vi "Process.vi"(8 "error in":errorcluster, 11 "Lockin.UI":refnum<class "Instrument.Lockin.UI.lvclass">) -> (0 "error out":errorcluster, 3 "Lockin.UI out":refnum<class "Instrument.Lockin.UI.lvclass">)   [LabVIEW 2016, in "Instrument.Lockin.UI.lvclass"]
doc: "---------------------------------------------------------------\nJKI State Machine Objects™\nhttp://jki.net/state-machine-objects/\nCopyright (C) 2005-2015, JKI <info@jki.net>\nALL RIGHTS RESERVEDJKI State Machine Objects (SMO) 1.0.0.5\nJKI - JKI\nCopyright (c) 2016, JKI"
uses:
  Instrument.Lockin.UI.lvclass
  <vilib>/JKI/JKI SMO/SMO/SMO.lvclass
  <vilib>/JKI/JKI SMO/SMO/Typedefs/Parent Call--Enum.ctl
  <vilib>/JKI/JKI SMO/SMO.UI/SMO.UI.lvclass
  <userlib>/LevyLab/Levylab Instruments/SMOs/Instrument/Instrument.lvclass
  Instrument.Lockin/Typedefs/Lockin.getAll--Cluster.ctl
  Instrument.Lockin/Instrument.Lockin.lvclass
  <userlib>/LevyLab/Levylab Instruments/SMOs/Instrument UI/Instrument UI.lvclass
  C:/Program Files (x86)/National Instruments/LabVIEW 2016/user.lib/LevyLab/Levylab Instruments/SMOs/Instrument UI/Instrument UI.lvclass
  C:/Program Files (x86)/National Instruments/LabVIEW 2016/vi.lib/JKI/JKI SMO/SMO.UI/SMO.UI.lvclass
  C:/Program Files (x86)/National Instruments/LabVIEW 2016/vi.lib/JKI/JKI SMO/SMO/SMO.lvclass
  Typedefs/Y Axis Input-Enum.ctl
  Typedefs/X Axis-Enum.ctl
  Typedefs/Y Axis Output-Enum.ctl
  Typedefs/Display-Enum.ctl
  Lockin.DAQ/Typedefs/Function-enum.ctl
  Lockin.DAQ/Lockin.DAQ.lvclass
  Lockin.DAQ/Typedefs/REF-cluster.ctl
  Lockin.DAQ/Typedefs/AI Simulation-enum.ctl
  Lockin.DAQ/Typedefs/DAQType-enum.ctl
  Lockin.DAQ/Typedefs/Sampling.ctl
  Instrument.Lockin/Typedefs/Sample Mode--Enum.ctl
  Lockin.DAQ/Typedefs/446xAI-enum.ctl
  Lockin.DAQ/Typedefs/AI.coupling-enum.ctl
  Lockin.DAQ/Typedefs/446xAO-enum.ctl
  Typedefs/Device Configuration--Cluster.ctl
  Lockin.DAQ/Typedefs/Sweep Pattern--Enum.ctl
  <vilib>/JKI/JKI SMO/SMO/Typedefs/SMOState --Enum.ctl
  Lockin.DAQ/Typedefs/Cal Info - Cluster.ctl
  Typedefs/AO Channel--Cluster.ctl
panel:
  out "Version":string="vDevelopment" caption="V"
  in  "Tab Control 4":T1(tab)
  in  "AO freq link":dbl=13.0 format="%.3p"
  in  "AO Amp Limit":dbl=0.009999999 format="%.3p"
  in  "Limit Amp":bool
  in  "Same f":bool
  in  "LP f (Hz)":dbl=100.0 format="%.3p"
  in  "Line":bool
  in  "Lowpass":bool
  in  "Measure":bool
  in  "Remove":bool
  in  "Channels: REF":T2={"Ch"=[1], " f (Hz)"=[13.0], "Phase (°)"=[0.0], "TC (s)"=[0.03], "order"=[2]} {"order" min=1; "TC (s)" min=0.0001 format="%#_3p"; "Phase (°)" format="%.3g"; "f (Hz)" format="%.3g"}
  in  "System Array":T3[](array[typedef]) {"REF.Ch 2" items=["1"]; "REF.Ch 1" items=["1"]; "Phase" format="%.3g"; "Frequency" min=0.0001 max=10000.0 format="%.3g"; "Offset" format="%.3p"; "Amplitude" min=0.0 max=10.0 format="%.3p"}
  in  "New Ch []":T5[](array[typedef]) {"AI.Coupling" items=["AC"=10045, "DC"=10050, "GND"=10066]}
  in  "auto DAQ":bool
  in  "Max Fs Refresh Rate (Hz)":dbl=10.0 format="%#_13g"
  in  "Sampling Mode":T9
  in  "Sampling":T10={"Fs"=10000.0, "#s"=1000}
  in  "DAQ Type":T11=enum."PXI 446x"
  in  "Auto x*F1":dbl=5000.0 format="%#_13g"
  in  "Load Configuration":bool
  in  "Save Configuration":bool
  in  "AI Simulation mode":T12=enum."AI = noise*AO"
  in  "decimating factor":i32=1
  in  "Update":bool
  in  "Enable Output":bool caption="Enable"
  in  "Input Channel":i32=1 min=1
  in  "input lockin result":enum16{"X", "Y", "R", "phi", "mean"}(ring)=enum."mean"
  in  "Output Channel":i32=1 min=1
  out "Output (V)":dbl
  in  "Aux Channel":tag="Dev2/ao0"
  in  "Voltage Output (V)":dbl min=-50.0 max=50.0
  in  "Amplifier Gain":dbl=1.0 min=-15.0 max=15.0
  out "DAQ Output (V)":dbl=-0.0 min=-3.5 max=3.5
  out "Amplified Output (V)":dbl=-0.0 min=-3.5 max=3.5
  in  "Pattern":T13[](array[typedef])=[enum."Ramp /"]
  in  "Step (V/update)":dbl=0.005 format="%#_6p"
  in  "Stop Sweep":bool caption="Stop"
  in  "Sweep Channel":u16[](array[ring])=[2] caption="Channel" items=["AO1"=1, "AO2"=2]
  in  "Sweep Start (V)":dbl[](array[numeric])=[0.0] caption="Start (V)" format="%#_6p"
  in  "Sweep End (V)":dbl[](array[numeric])=[0.1] caption="End (V)" format="%#_6p"
  in  "Sweep Time (s)":dbl=20.0 format="%#_1f"
  in  "Start Sweep":bool caption="Start"
  in  "Initial Wait (s)":dbl=1.0
  out "Sweep Timer (s)":dbl caption="Timer (s)"
  in  "Return to Start?":bool
  out "Sampling Status":string="Good"
  in  "Output Gain":cluster{"AI.Ch":string, "Gain":dbl}[](array[cluster])=[{"AI.Ch"="AO1", "Gain"=1.0}, {"AI.Ch"="AO2", "Gain"=1.0}, {"AI.Ch"="AO3", "Gain"=1.0}, {"AI.Ch"="AO4", "Gain"=1.0}, {"AI.Ch"="AO5", "Gain"=1.0}, {"AI.Ch"="AO6", "Gain"=1.0}, {"AI.Ch"="AO7", "Gain"=1.0}, {"AI.Ch"="AO8", "Gain"=1.0}, {"AI.Ch"="AO9", "Gain"=1.0}, {"AI.Ch"="AO10", "Gain"=1.0}, {"AI.Ch"="AO11", "Gain"=1.0}, {"AI.Ch"="AO12", "Gain"=1.0}, {"AI.Ch"="AO13", "Gain"=1.0}, {"AI.Ch"="AO14", "Gain"=1.0}, {"AI.Ch"="AO15", "Gain"=1.0}, {"AI.Ch"="AO16", "Gain"=1.0}]
  in  "Input Gain":cluster{"AI.Ch":string, "Gain":dbl}[](array[cluster])=[{"AI.Ch"="AI1", "Gain"=1.0}, {"AI.Ch"="AI2", "Gain"=1.0}, {"AI.Ch"="AI3", "Gain"=1.0}, {"AI.Ch"="AI4", "Gain"=1.0}, {"AI.Ch"="AI5", "Gain"=1.0}, {"AI.Ch"="AI6", "Gain"=1.0}, {"AI.Ch"="AI7", "Gain"=1.0}, {"AI.Ch"="AI8", "Gain"=1.0}, {"AI.Ch"="AI9", "Gain"=1.0}, {"AI.Ch"="AI10", "Gain"=1.0}, {"AI.Ch"="AI11", "Gain"=1.0}, {"AI.Ch"="AI12", "Gain"=1.0}, {"AI.Ch"="AI13", "Gain"=1.0}, {"AI.Ch"="AI14", "Gain"=1.0}, {"AI.Ch"="AI15", "Gain"=1.0}, {"AI.Ch"="AI16", "Gain"=1.0}]
  out "State History":string=" Exit\r Data: Cleanup\r Events: Unregister\r UI: Cleanup\r UI: Disable Buttons\r Configuration: Write\r Error Logger: Destroy\r Lockin SMO: Stop\r Remote SMO: Stop\r Macro: Exit\r UI: Update Sweep Timer\r UI: Update Lockin Graphs\r UI: Update Waveform Graphs\r 4461: OUT\r UI: Update Sweep Timer\r UI: Update Lockin Graphs\r UI: Update Waveform Graphs\r 4461: OUT\r UI: Update Sweep Timer\r UI: Update Lockin Graphs\r UI: Update Waveform Graphs\r 4461: OUT"
  out "Refresh time (ms)":u32=103
  out "LockinDAQ SMO State":T14=enum."Stopped" caption="SMO State"
  out "RC SMO State":T14=enum."Stopped" caption="SMO State"
  in  "Allowed remote system":string
  in  "Get Calibration":bool
  out "Cal Info":T15[](array[typedef]) {"SelfCal.LastDate/Time" format="%<%I:%M %p\n%m/%d/%Y>T"}
  in  "Self Calibrate":bool
  in  "Save":bool
  in  "Path":path=path "C:/Data/lockin"
  in  "Notes":string
  in  "Tab Control 3":enum32{"Page 1"}(tab)
  in  "Channel":u16(ring)=1 items=["AI1 f1 (0.0 Hz)"=1, "AI2 f1 (0.0 Hz)"=2]
  out "X":dbl=0.0014996100939563214 caption="Magnitude (V)" format="%#_3p"
  out "Y":dbl=-29.79492153733761 caption="Phase (°)" format="%#_3p"
  in  "Display":T16=enum."R and Theta" caption="Enum"
  in  "Close":bool
  out "Status":string="Shutdown"
  in  "Pause":bool
  in  "Reset":bool
  in  "Start":bool
  in  "Help":bool
  in  "Trigger":bool
  in  "Tab Control 2":T17(tab)
  in  "Decimate":enum16{"1", "10", "100", "1000"}(ring) caption="Enum"
  in  "Y Axis Output":T18 caption="Enum"
  in  "X Axis":T19 caption="Enum"
  in  "Y Axis Input":T20 caption="Enum"
  out "Input Graph":waveform(dbl)[](graph)
  out "Output Graph":waveform(dbl)[](graph)
  in  "YorTheta Axis Range":dbl=180.0 caption="Axis Range" format="%#_6p"
  in  "XorR Axis Range":dbl=0.0001 caption="Axis Range" format="%#_6p"
  out "Lockin Display 2":waveform(dbl)[](graph)=[{"t0"=timestamp(3696860787.849275 s since 1904-01-01), "dt"=1.0, "Y"=[-29.79492153733761]}, {"t0"=timestamp(3696860787.849275 s since 1904-01-01), "dt"=1.0, "Y"=[79.44593778514711]}, {"t0"=timestamp(3696860787.849275 s since 1904-01-01), "dt"=1.0, "Y"=[143.51884004503978]}, {"t0"=timestamp(3696860787.849275 s since 1904-01-01), "dt"=1.0, "Y"=[176.51469468021597]}, {"t0"=timestamp(3696860787.849275 s since 1904-01-01), "dt"=1.0, "Y"=[-53.240868302891855]}, {"t0"=timestamp(3696860787.849275 s since 1904-01-01), "dt"=1.0, "Y"=[129.5970530362907]}, {"t0"=timestamp(3696860787.849275 s since 1904-01-01), "dt"=1.0, "Y"=[34.65839026734602]}, {"t0"=timestamp(3696860787.849275 s since 1904-01-01), "dt"=1.0, "Y"=[-148.74995852714687]}, {"t0"=timestamp(3696860787.849275 s since 1904-01-01), "dt"=1.0, "Y"=[-78.04356650876782]}, {"t0"=timestamp(3696860787.849275 s since 1904-01-01), "dt"=1.0, "Y"=[-149.42192221469682]}, {"t0"=timestamp(3696860787.849275 s since 1904-01-01), "dt"=1.0, "Y"=[-10.103060653866786]}, {"t0"=timestamp(3696860787.849275 s since 1904-01-01), "dt"=1.0, "Y"=[139.82545965539245]}, {"t0"=timestamp(3696860787.849275 s since 1904-01-01), "dt"=1.0, "Y"=[165.6018484082086]}, {"t0"=timestamp(3696860787.849275 s since 1904-01-01), "dt"=1.0, "Y"=[156.22326907992732]}, {"t0"=timestamp(3696860787.849275 s since 1904-01-01), "dt"=1.0, "Y"=[35.00025461826527]}, {"t0"=timestamp(3696860787.849275 s since 1904-01-01), "dt"=1.0, "Y"=[-137.0348206815793]}]
  out "Lockin Display 1":waveform(dbl)[](graph)=[{"t0"=timestamp(3696860787.849275 s since 1904-01-01), "dt"=1.0, "Y"=[0.0014996100939563214]}, {"t0"=timestamp(3696860787.849275 s since 1904-01-01), "dt"=1.0, "Y"=[0.0011784669494735013]}, {"t0"=timestamp(3696860787.849275 s since 1904-01-01), "dt"=1.0, "Y"=[0.002904634901901364]}, {"t0"=timestamp(3696860787.849275 s since 1904-01-01), "dt"=1.0, "Y"=[0.0016663260472614767]}, {"t0"=timestamp(3696860787.849275 s since 1904-01-01), "dt"=1.0, "Y"=[0.0017826595136042982]}, {"t0"=timestamp(3696860787.849275 s since 1904-01-01), "dt"=1.0, "Y"=[0.0016963363783871741]}, {"t0"=timestamp(3696860787.849275 s since 1904-01-01), "dt"=1.0, "Y"=[0.0006272329797125746]}, {"t0"=timestamp(3696860787.849275 s since 1904-01-01), "dt"=1.0, "Y"=[0.0010044050863696411]}, {"t0"=timestamp(3696860787.849275 s since 1904-01-01), "dt"=1.0, "Y"=[0.0036270540010642054]}, {"t0"=timestamp(3696860787.849275 s since 1904-01-01), "dt"=1.0, "Y"=[0.002787136933442983]}, {"t0"=timestamp(3696860787.849275 s since 1904-01-01), "dt"=1.0, "Y"=[0.0020988006734285343]}, {"t0"=timestamp(3696860787.849275 s since 1904-01-01), "dt"=1.0, "Y"=[0.0025753210454415427]}, {"t0"=timestamp(3696860787.849275 s since 1904-01-01), "dt"=1.0, "Y"=[0.001463110575523916]}, {"t0"=timestamp(3696860787.849275 s since 1904-01-01), "dt"=1.0, "Y"=[0.00358223110996865]}, {"t0"=timestamp(3696860787.849275 s since 1904-01-01), "dt"=1.0, "Y"=[0.002881444954025323]}, {"t0"=timestamp(3696860787.849275 s since 1904-01-01), "dt"=1.0, "Y"=[0.0005817216121370231]}]
  in  "X&Y Axis Range":dbl=1e-06 caption="Numeric" format="%#_6p"
  out "XY Graph":cluster{dbl[], dbl[]}[](graph)=[{[0.0, 0.0013013758853688236], [0.0, -0.0007451518227020566]}, {[0.0, 0.0002158517867763353], [0.0, 0.0011585302573290193]}, {[0.0, -0.0023354786851164104], [0.0, 0.0017269751662112775]}, {[0.0, -0.0016632440485085782], [0.0, 0.000101300201790775]}, {[0.0, 0.0010668366777369248], [0.0, -0.0014281927196562634]}, {[0.0, -0.0010812182737586773], [0.0, 0.0013071052570967727]}, {[0.0, 0.000515935035064585], [0.0, 0.0003566962999976595]}, {[0.0, -0.0008586774541396104], [0.0, -0.0005210591207123463]}, {[0.0, 0.0007514090440462253], [0.0, -0.0035483665502821717]}, {[0.0, -0.002399548559736948], [0.0, -0.0014178501314406596]}, {[0.0, 0.002066256272976915], [0.0, -0.0003681701796284117]}, {[0.0, -0.0019677584263203063], [0.0, 0.0016613865482600827]}, {[0.0, -0.0014171560040281868], [0.0, 0.0003638150855266809]}, {[0.0, -0.003278183803234751], [0.0, 0.001444261291261581]}, {[0.0, 0.002360334179965922], [0.0, 0.001652739417440812]}, {[0.0, -0.0004256852846233785], [0.0, -0.0003964745546468404]}]
  out "Results (X, Y, R, Theta, mean)":dbl[][](array[numeric])=[[0.0013013758853688236, -0.0007451518227020566, 0.0014996100939563214, -29.79492153733761, 0.0013487518998213243], [0.0002158517867763353, 0.0011585302573290193, 0.0011784669494735013, 79.44593778514711, -0.0026309333585394406], [-0.0023354786851164104, 0.0017269751662112775, 0.002904634901901364, 143.51884004503978, 0.00033634501962841325], [-0.0016632440485085782, 0.000101300201790775, 0.0016663260472614767, 176.51469468021597, 0.001631642536934811], [0.0010668366777369248, -0.0014281927196562634, 0.0017826595136042982, -53.240868302891855, 0.0022470560632466235], [-0.0010812182737586773, 0.0013071052570967727, 0.0016963363783871741, 129.5970530362907, 0.0030006354378964337], [0.000515935035064585, 0.0003566962999976595, 0.0006272329797125746, 34.65839026734602, 0.0037885404293860818], [-0.0008586774541396104, -0.0005210591207123463, 0.0010044050863696411, -148.74995852714687, 0.00041948801212486126], [0.0007514090440462253, -0.0035483665502821717, 0.0036270540010642054, -78.04356650876782, -0.0006792110611968232], [-0.002399548559736948, -0.0014178501314406596, 0.002787136933442983, -149.42192221469682, -0.002735327879128451], [0.002066256272976915, -0.0003681701796284117, 0.0020988006734285343, -10.103060653866786, -0.0007457891804275254], [-0.0019677584263203063, 0.0016613865482600827, 0.0025753210454415427, 139.82545965539245, -0.003081895874292059], [-0.0014171560040281868, 0.0003638150855266809, 0.001463110575523916, 165.6018484082086, -0.003651412270249597], [-0.003278183803234751, 0.001444261291261581, 0.00358223110996865, 156.22326907992732, -0.0003916792750837599], [0.002360334179965922, 0.001652739417440812, 0.002881444954025323, 35.00025461826527, -0.0017434733726545428], [-0.0004256852846233785, -0.0003964745546468404, 0.0005817216121370231, -137.0348206815793, -0.001062718455061755]] format="%.3p"
  out "Sweep X WFMs":waveform(dbl)[](graph)
  out "Sweep Y WFMs":waveform(dbl)[](graph)
  out "Sweep AI WFMs":waveform(dbl)[](graph)
  out "Sweep AO WFMs":waveform(dbl)[](graph)
  in  "number of averages":u32=10 min=1
  in  "weighting mode":enum16{"Linear", "Exponential"}(ring)=enum."Exponential"
  in  "averaging mode":T21(ring)=enum."RMS averaging"
  in  "window":u16(ring) items=["Rectangle", "Hanning"]
  in  "export mode":u16(ring)=1 items=["Power Spectrum", "Power Spectral Density"]
  in  "restart averaging":bool
  out "averaging done?":bool=TRUE
  out "PS Chart":dbl[][](graph)=[[-1266.4439057806233, -1267.126235485124, -1268.7165302459164, -1271.0871036455492, -1261.5500005179456, -1261.6863547163412]]
  out "PS dB":cluster{"f0":dbl, "df":dbl, "magnitude":dbl[]}[](graph)
  out "averages completed":dbl=180.0
  in  "STOP":bool
  # "v2020/03/13 v2.9.10"
  # "Lockin UI"
  # "For instructions on how to use the JKI State Machine Objects, examples and video tutorials, visit:\nhttp://jki.net/state-machine-objects/\n\nJKI State Machine Objects™\nhttp://jki.net/state-machine-objects/\nCopyright (C) 2005-2015, JKI <info@jki.net>\nALL RIGHTS RESERVED"
  # "Output"
  # "Input: Pre-Filter"
  # "Input: Offset"
  # "Reference"
  # "TC and order are the same for all Reference channels"
  # "DAQ Channels"
  # "Device"
  # "AI.Ch"
  # "AI.Range"
  # "AI.Coupling"
  # "AO.Ch"
  # "AO.Range"
  # "LIA.Ch"
  # "Configuration"
  # "Sampling"
  # "Changing settings in this box will automatically\nreset the lockin and restart acquisition"
  # "Auxiliary Output"
  # "Configuration"
  # "- Use to control an auxiliiary card such as a multifunction DAQ (6115, 6120, etc)"
  # "Forward Lockin Input --> Lockin Output"
  # "- Choose an input lockin channel and value (X,Y, etc) and it will be written as a DC value to an output channel of your choosing.\n- Output is scaled by the input amplifier gain."
  # "Sweep"
  # "Status"
  # "Channel"
  # "Channel"
  # "Input Gain"
  # "Output Gain"
  # "Calibration"
  # "Self Cal\nLast Time"
  # "Self Cal\nLast Temp"
  # "Temp\nNow"
  # "Cal\nDue"
  # "Device"
  # "AO/AI Display"
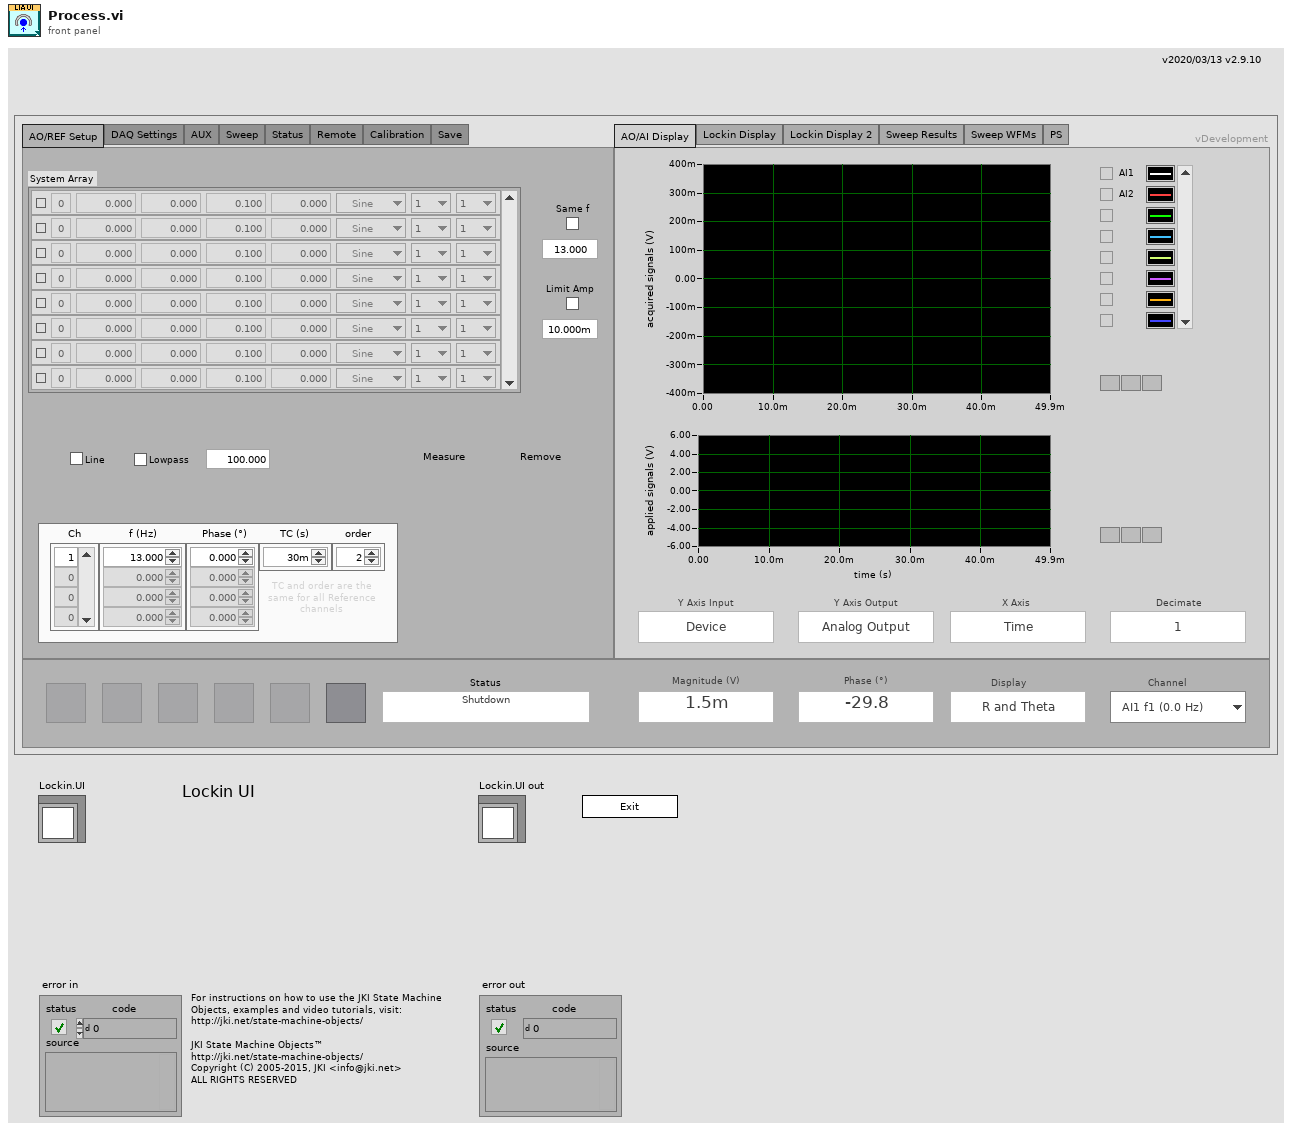
[diagram p1: front panel]
types:
  T1 = enum32{"AO/REF Setup", "DAQ Settings", "AUX", "Sweep", "Status", "Remote", "Calibration", "Save"}
  T2 = typedef "Lockin.DAQ.lvclass/REF-cluster.ctl" = cluster{"Ch":i32[], " f (Hz)":dbl[], "Phase (°)":dbl[], "TC (s)":dbl[], "order":i32[]}
  T3 = typedef "Instrument.Lockin.UI.lvclass/AO Channel--Cluster.ctl" = cluster{"Channel":i32, "Amplitude":dbl, "Offset":dbl, "Frequency":dbl, "Phase":dbl, "Function":T4, "Sweeping?":bool, "REF.Ch 1":u16, "REF.Ch 2":u16}
  T4 = typedef "Lockin.DAQ.lvclass/Function-enum.ctl" = enum16{"Sine", "Triangle", "Square"}
  T5 = typedef "Instrument.Lockin.UI.lvclass/Device Configuration--Cluster.ctl" = cluster{"Device":string, "AI.Ch":string, "AI.Range":T6, "AI.Coupling":T7, "AO.Ch":string, "AO.Range":T8}
  T6 = typedef "Lockin.DAQ.lvclass/446xAI-enum.ctl" = enum16{"±0.316", "±1.00", "±3.16", "±10.0", "±31.6", "±42.4"}
  T7 = typedef "Lockin.DAQ.lvclass/AI.coupling-enum.ctl" = u16
  T8 = typedef "Lockin.DAQ.lvclass/446xAO-enum.ctl" = enum16{"±0.1", "±1.0", "±10.0"}
  T9 = typedef "Instrument.Lockin.lvclass/Sample Mode--Enum.ctl" = enum16{"Manual", "Auto Fs", "Max Fs"}
  T10 = typedef "Lockin.DAQ.lvclass/Sampling.ctl" = cluster{"Fs":dbl, "#s":i32}
  T11 = typedef "Lockin.DAQ.lvclass/DAQType-enum.ctl" = enum16{"None", "USB 4431", "PXI 446x"}
  T12 = typedef "Lockin.DAQ.lvclass/AI Simulation-enum.ctl" = enum16{"AI = HW simulated", "AI = noise*AO", "AI = waveguide"}
  T13 = typedef "Lockin.DAQ.lvclass/Sweep Pattern--Enum.ctl" = enum16{"Ramp /", "Ramp /\\", "Smooth Ramp _/", "Smooth Ramp _/\\_", "Frequency"}
  T14 = typedef "SMO.lvclass/SMOState --Enum.ctl" = enum16{"unknown", "Created", "Started", "Stopped"}
  T15 = typedef "Lockin.DAQ.lvclass/Cal Info - Cluster.ctl" = cluster{"Active Device":string, "SelfCal.LastDate/Time":dbl, "SelfCal.LastTemp":dbl, "DevTemp":dbl, "calibration due?":bool}
  T16 = typedef "Instrument.Lockin.UI.lvclass/Display-Enum.ctl" = enum16{"X and Y", "R and Theta"}
  T17 = enum32{"AO/AI Display", "Lockin Display", "Lockin Display 2", "Sweep Results", "Sweep WFMs", "PS"}
  T18 = typedef "Instrument.Lockin.UI.lvclass/Y Axis Output-Enum.ctl" = enum16{"Analog Output", "Reference"}
  T19 = typedef "Instrument.Lockin.UI.lvclass/X Axis-Enum.ctl" = enum16{"Time", "Samples"}
  T20 = typedef "Instrument.Lockin.UI.lvclass/Y Axis Input-Enum.ctl" = enum16{"Device", "ADC"}
  T21 = enum16{"No averaging", "Vector averaging", "RMS averaging", "Peak hold"}
  T22 = typedef "SMO.lvclass/Parent Call--Enum.ctl" = enum16{"Allows parent to run", "Does not request parent to run"}
  T23 = enum32{"invalid app kind", "Development System", "Run Time System", "Student Edition", "Embedded LabVIEW", "Evaluation", "Custom"}
  T24 = enum32{"Invalid", "Standard", "Closed", "Hidden", "Minimized", "Maximized"}
  T25 = typedef "Instrument.Lockin.lvclass/Lockin.getAll--Cluster.ctl" = cluster{"Not Supported":string}
  T26 = cluster{"Current VI Reference":refnum<vi>, "Close Panel on Exit?":bool, "error":errorcluster}
  T27 = cluster{"Core":cluster{"Current VI Reference":refnum<vi>, "Close Panel on Exit?":bool, "error":errorcluster}, "Self Reference":refnum<class "Instrument.Lockin.UI.lvclass">, "Instrument":refnum<class "Instrument.lvclass">, "getAll":variant, void}
  T28 = typedef "SMO.lvclass/Protected Events.ctl" = cluster{"StopProcesses":refnum<user-event>, "AbortProcesses":refnum<user-event>, "Config Changed":refnum<user-event>, "Dependency":refnum<user-event>}
  T29 = typedef "Instrument.lvclass/PublicEvents--Cluster.ctl" = cluster{"MessageFromProcess":refnum<user-event>}
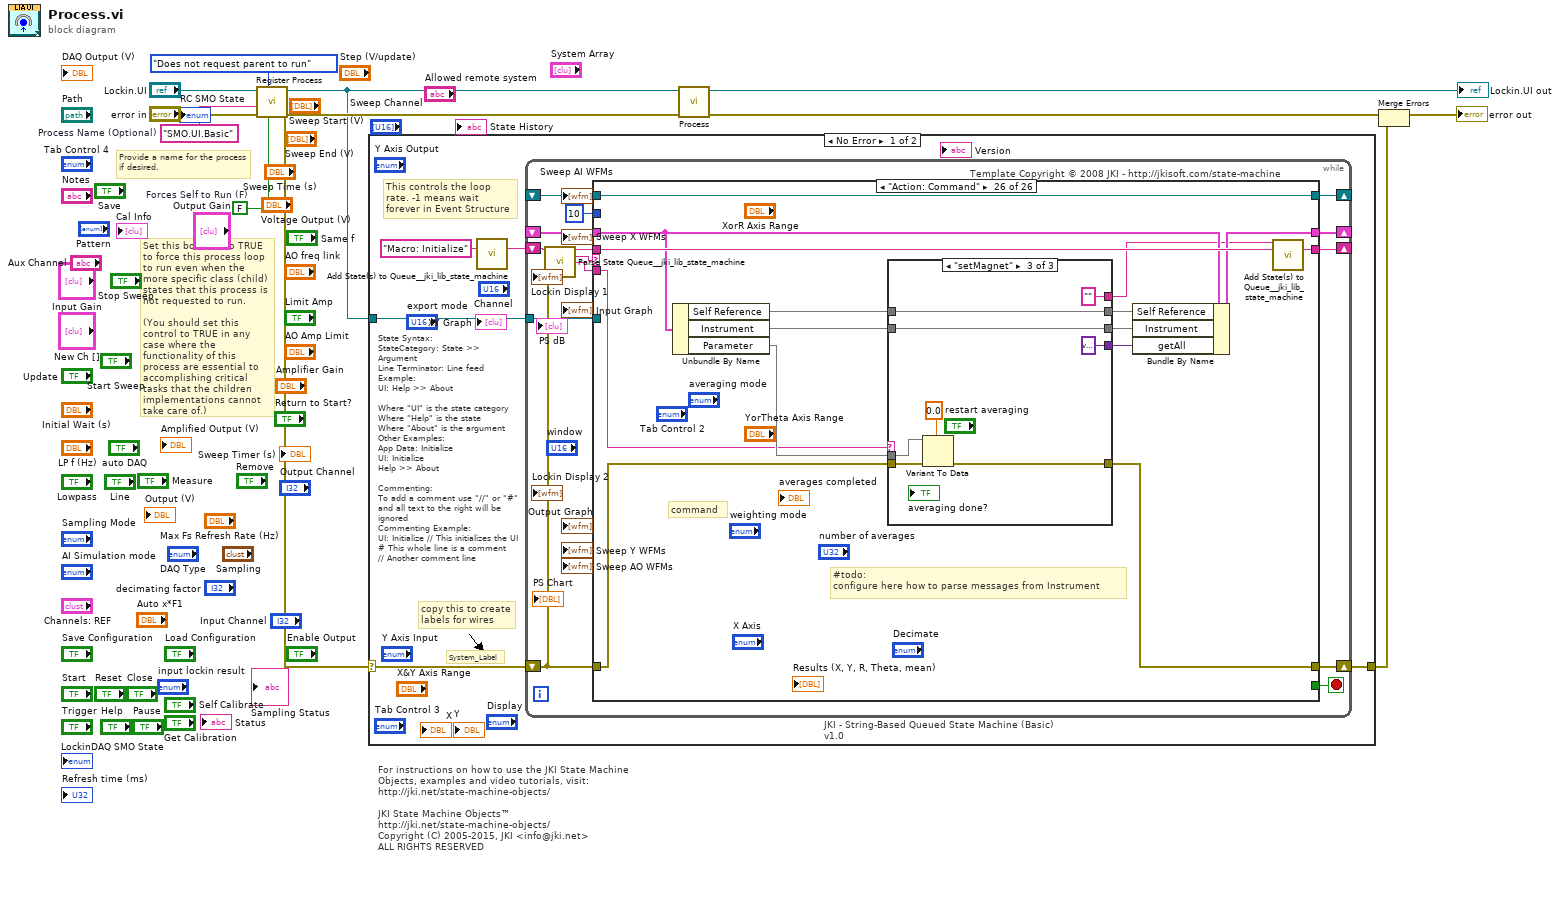
[diagram p0: block diagram]
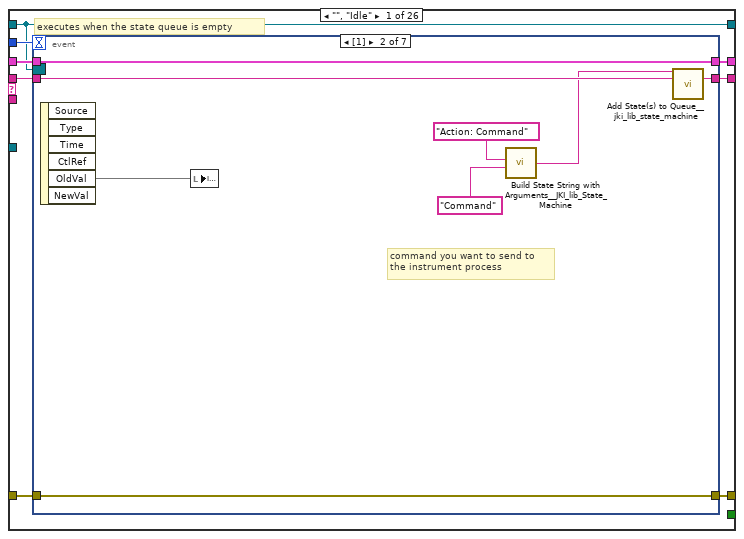
[diagram p2: hidden frame]
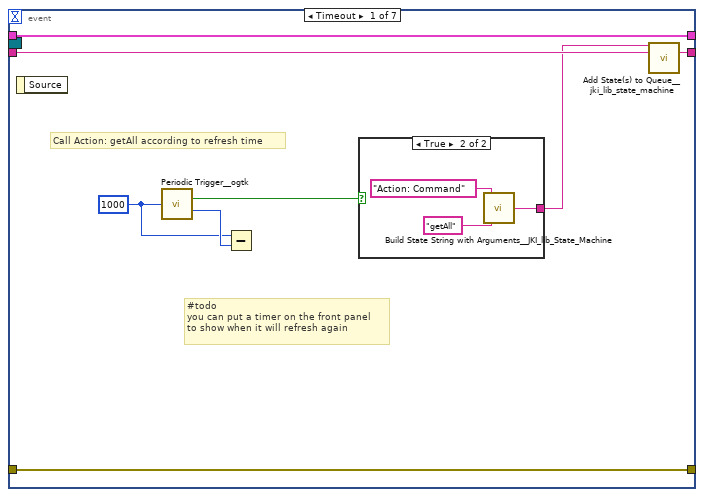
[diagram p3: hidden frame]
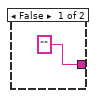
[diagram p4: hidden frame]
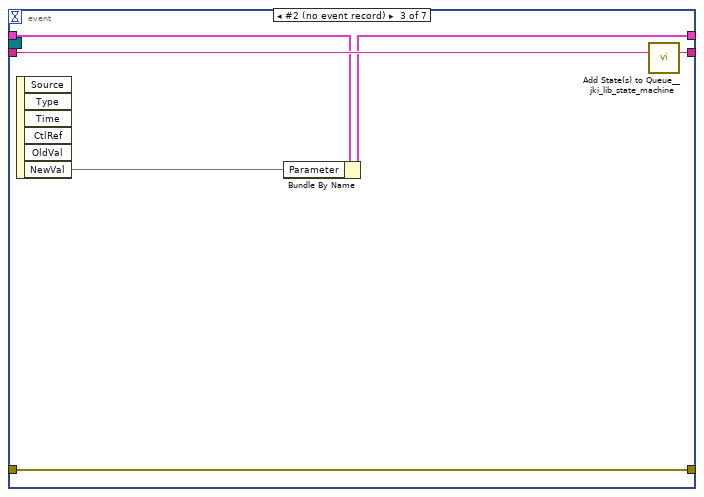
[diagram p5: hidden frame]
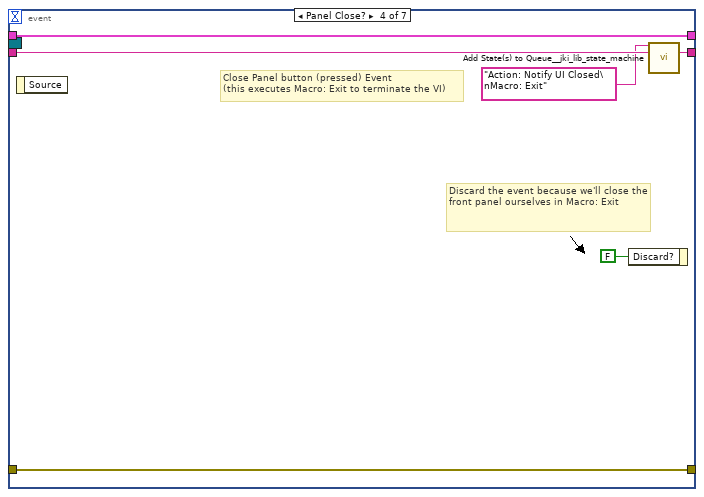
[diagram p6: hidden frame]
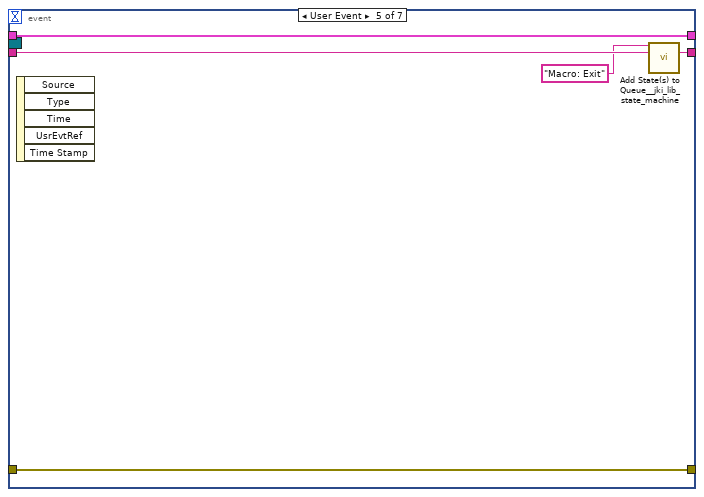
[diagram p7: hidden frame]
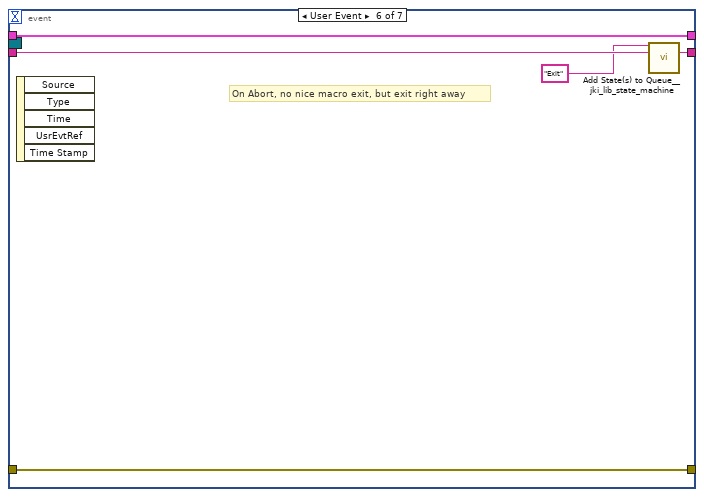
[diagram p8: hidden frame]
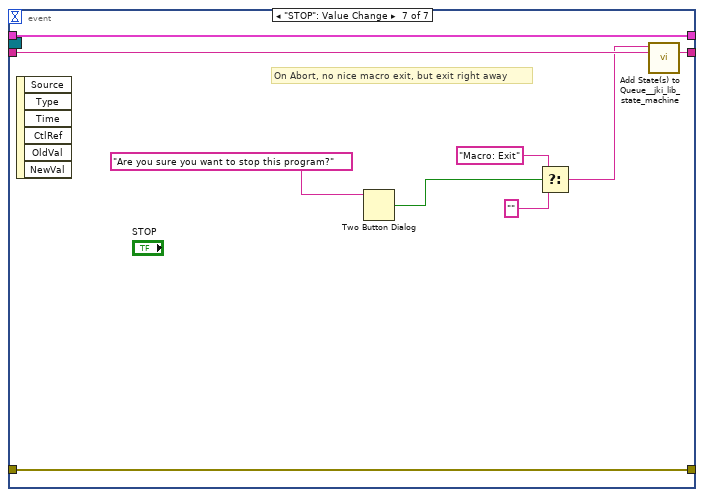
[diagram p9: hidden frame]
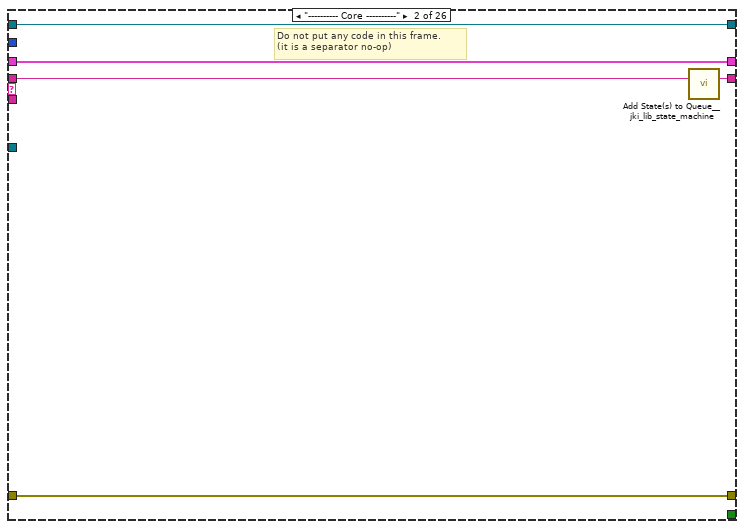
[diagram p10: hidden frame]
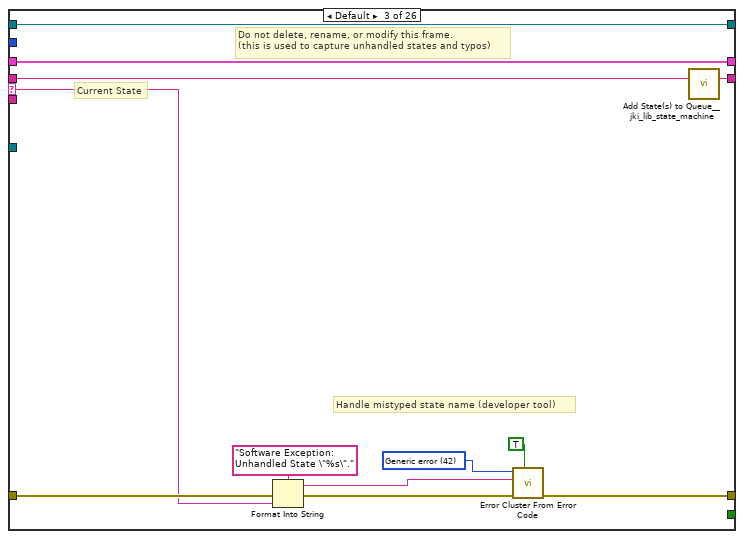
[diagram p11: hidden frame]
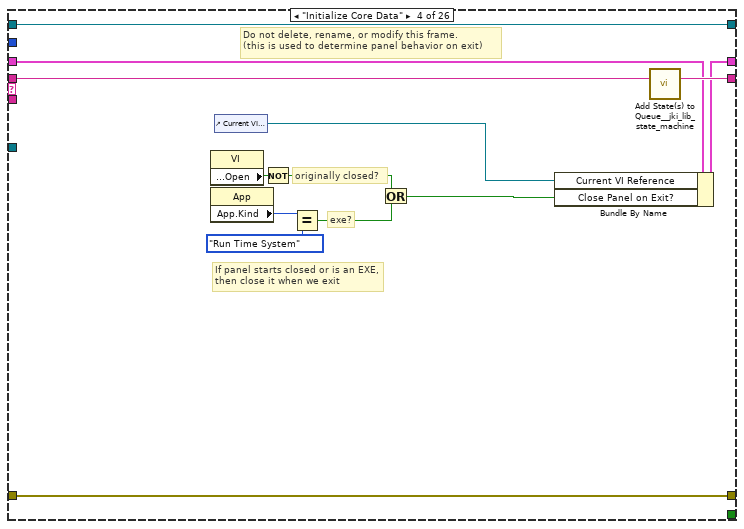
[diagram p12: hidden frame]
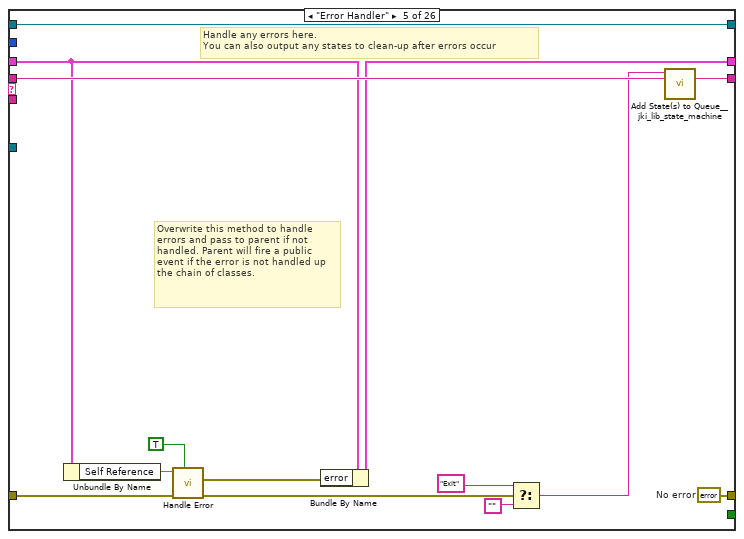
[diagram p13: hidden frame]
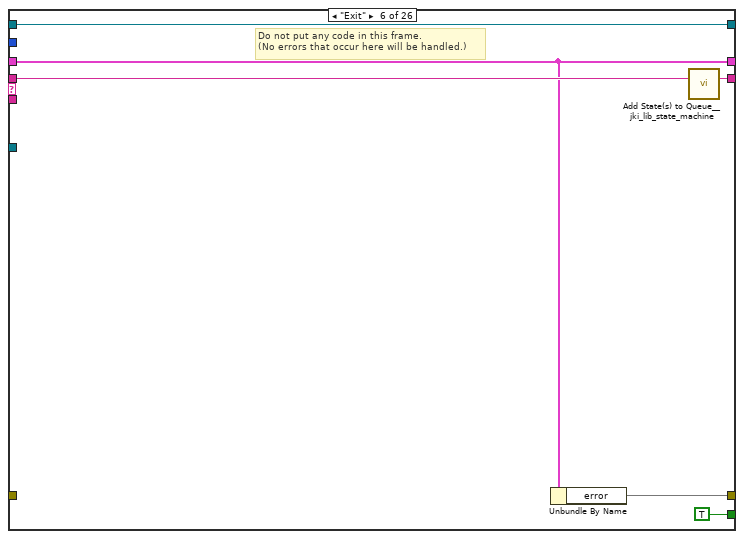
[diagram p14: hidden frame]
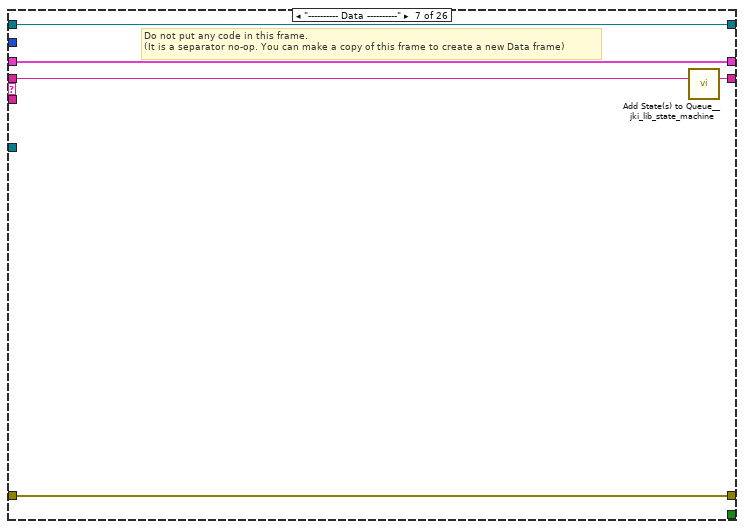
[diagram p15: hidden frame]
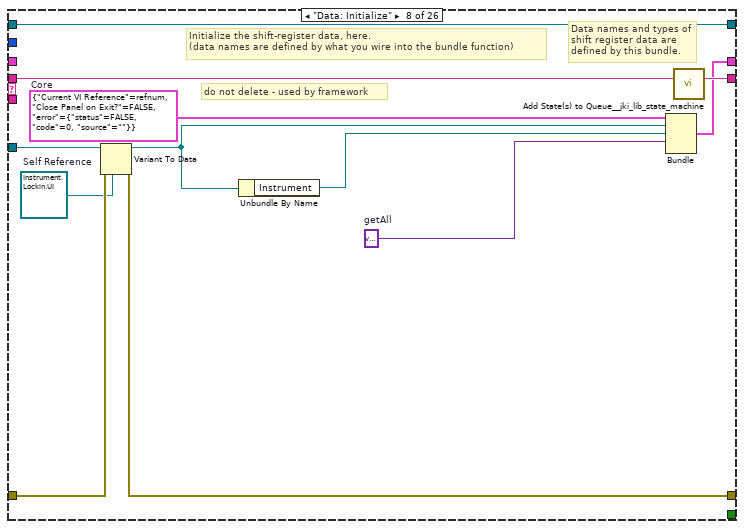
[diagram p16: hidden frame]
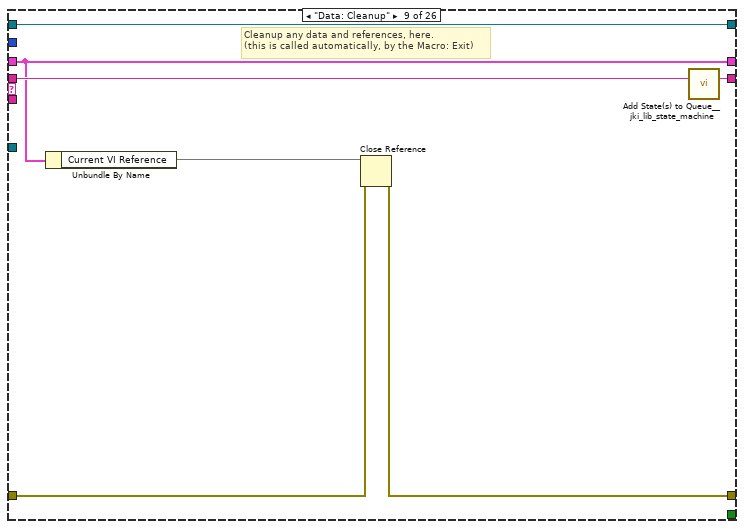
[diagram p17: hidden frame]
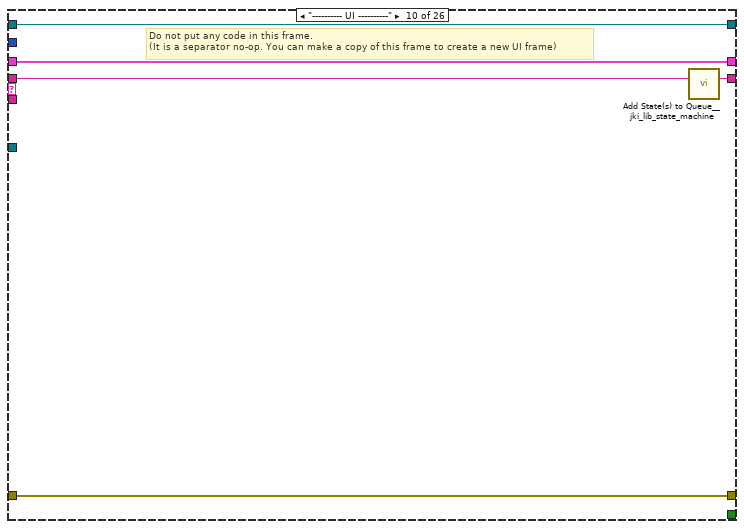
[diagram p18: hidden frame]
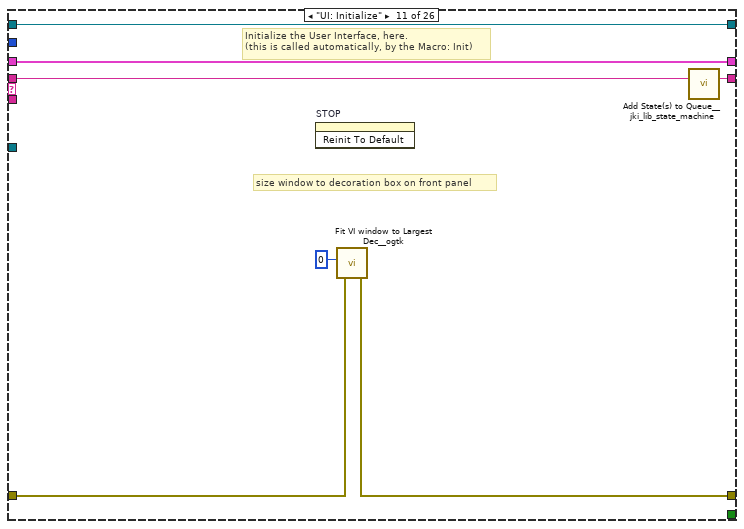
[diagram p19: hidden frame]
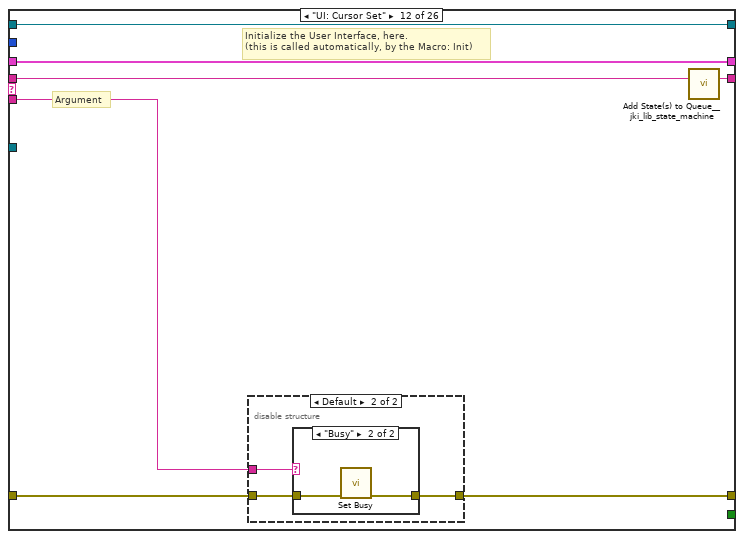
[diagram p20: hidden frame]
diagram:
  w2 = FALSE  # Forces Self to Run (F)
  w1 = "SMO.UI.Basic"  # Process Name (Optional)
  # "Provide a name for the process\nif desired."
  # "Set this boolean to TRUE to force this process loop to run even when the more specific class (child) states that this process is not requested to run.\n\n(You should set this control to TRUE in any case where the functionality of this process are essential to accomplishing critical tasks that the children implementations cannot take care of.)"
  # "For instructions on how to use the JKI State Machine Objects, examples and video tutorials, visit:\nhttp://jki.net/state-machine-objects/\n\nJKI State Machine Objects™\nhttp://jki.net/state-machine-objects/\nCopyright (C) 2005-2015, JKI <info@jki.net>\nALL RIGHTS RESERVED"
  n1 = call <vilib>:"Register Process.vi"("Forces Self to Run (F)"=w2, "Parent Call"=Parent_Call--Enum."Does not request parent to run", "error in (no error)"="error in", "Process Name (optional)"=w1, "SMO"="Lockin.UI") -> ("error out"=w8:errorcluster, "SMO out"=w7:refnum<class "Instrument.Lockin.UI.lvclass">)  [unwired: 5 in]
  n2 = case shown="No Error" w8 {
    selector: w8 -> [w13 w361]
    tunnel: w7 -> [w14 _]
    tunnel: [w12 w361] -> w4
    frame No Error {
      # "State Syntax:\nStateCategory: State >> Argument\nLine Terminator: Line feed\nExample:\nUI: Help >> About\n\nWhere \"UI\" is the state category\nWhere \"Help\" is the state\nWhere \"About\" is the argument\nOther Examples:\nApp Data: Initialize\nUI: Initialize\nHelp >> About\n\nCommenting:\nTo add a comment use \"//\" or \"#\" and all text to the right will be ignored\nCommenting Example:\nUI: Initialize // This initializes the UI\n# This whole line is a comment\n// Another comment line"
      # "copy this to create labels for wires"
      # "This controls the loop rate. -1 means wait forever in Event Structure"
      # "System_Label"
      n3 = call <vilib>:"Add State(s) to Queue__jki_lib_state_machine.vi"("State(s) in (\"\")"="Macro: Initialize") -> ("States Out"=w16:string)  [unwired: 14 in]
      n4 = while "JKI - String-Based Queued State Machine (Basic) v1.0" {
        shift-right: [w23] -> _
        shift-left: _ -> [w22]
        shift-right: [w26] -> w12
        shift-left: w13 -> [w20]
        shift-right: [w25] -> _
        shift-left: w16 -> [w27]
        tunnel: w14 -> [w19]
        shift-right: [w18] -> _
        shift-left: _ -> [w17]
        stop <- w24 stop-if-true
        # "Template Copyright © 2008 JKI - http://jkisoft.com/state-machine"
        n5 = call <vilib>:"Parse State Queue__jki_lib_state_machine.vi"("State Queue"=w27, "Error In (no error)"=w20) -> ("Remaining States"=w29:string, "Current State"=w30:string, "Arguments"=w28:string)  [unwired: 11 in]
        n6 = case shown="\"Action: Command\"" w30 {
          selector: w30 -> [_ _ w97 _ _ _ _ _ _ _ _ _ _ _ _ _ _ _ _ _ _ _ _ _ _ _]
          tunnel: w29 -> [w38 w95 w101 w120 w134 w140 w145 w158 w165 w170 w177 w184 w200 w232 w241 w255 w260 w271 w278 w283 w296 w302 w309 w316 w326 w341]
          tunnel: w28 -> [_ _ _ _ _ _ _ _ _ _ _ w178 w194 _ _ _ _ _ _ _ _ _ _ _ _ w333]
          tunnel: w22 -> [w36 w92 w99 w111 w123 w136 w142 _ w160 w167 w175 w182 w196 w229 w237 w246 w257 w268 w273 w280 w294 w300 w305 w312 w323 w338]
          tunnel: [w35 w93 w103 w117 w125 w135 w143 w154 w161 w168 w172 w179 w197 w230 w239 w253 w258 w262 w274 w281 w289 w297 w306 w310 w319 w334] -> w26
          tunnel: w20 -> [w34 w93 w102 w117 w130 _ w143 w155 w162 w168 w173 w180 w198 w230 w239 w253 w258 w263 w275 w281 w291 w298 w306 w311 w320 w335]
          tunnel: [w37 w94 w100 w119 w133 w139 w144 w157 w164 w169 w176 w183 w199 w231 w240 w254 w259 w270 w277 w282 w295 w301 w308 w315 w325 w340] -> w25
          tunnel: [_ _ _ _ _ TRUE _ _ _ _ _ _ _ _ _ _ _ _ _ _ _ _ _ _ _ _] -> w24
          tunnel: [w33 w92 w99 w118 w122 w136 w142 w156 w160 w167 w175 w182 w196 w229 w237 w246 w257 w268 w273 w280 w294 w300 w304 w312 w323 w337] -> w23
          tunnel: 10 ("Timeout") -> [w32 _ _ _ _ _ _ _ _ _ _ _ _ _ _ _ _ _ _ _ _ _ _ _ _ _]
          tunnel: w19 -> [_ _ _ _ _ _ _ w152 _ _ _ _ _ _ _ _ _ _ _ _ _ _ _ _ _ _]
          tunnel: [w31 w91 w96 w108 w132 w137 w141 w151 w159 w166 w174 w181 w193 w228 w238 w247 w256 w269 w276 w279 w293 w299 w307 w314 w324 w339] -> w18
          tunnel: w17 -> [w31 w91 w96 w108 w132 w137 w141 w151 w159 w166 w174 w181 w193 w228 w238 w247 w256 w269 w276 w279 _ w299 w307 w314 w324 w339]
          frame "", "Idle" {
            # "executes when the state queue is empty"
            n7 = event shown="[1]" {
              selector: w31 -> [_ _ _ _ _ _ _]
              dyn-events: _ -> [_ _ _ _ _ _ _]
              timeout: w32 -> [_ _ _ _ _ _ _]
              tunnel: w38 -> [w47 w59 w65 w71 w76 w81 w90]
              tunnel: [w46 w58 w64 w70 w75 w80 w89] -> w37
              tunnel: w36 -> [w44 w56 w61 w67 w73 w78 w87]
              tunnel: [w45 w57 w63 w66 w74 w79 w88] -> w35
              tunnel: w34 -> [w45 w57 w63 w66 w74 w79 w88]
              tunnel: [w44 w56 w60 w67 w73 w78 w87] -> w33
              event Timeout {
                w39 = u32 1000 ("time (ms)")
                # "#todo\nyou can put a timer on the front panel\nto show when it will refresh again"
                # "Call Action: getAll according to refresh time"
                n8 = event-data() -> ()  [unwired: 1 in, 1 out]
                n9 = call <userlib>:"Periodic Trigger__ogtk.vi"("time (ms)"=w39) -> ("Triggered"=w42:bool, "timer value"=w40:u32)  [unwired: 12 in, 1 out]
                n10 = Subtract(x=w39, y=w40) -> (x-y=w41:u32)
                n11 = case shown="True" w42 {
                  tunnel: ["" ("State(s) in Front (\"\")") w49] -> w43
                  frame False {
                  }
                  frame True {
                    n12 = call <vilib>:"Build State String with Arguments__JKI_lib_State_Machine.vi"("Arguments (\"\")"="getAll" ("State(s) in Front (\"\")"), "State"="Action: Command" ("State(s) in Front (\"\")")) -> ("State with Arguments"=w49:string)  [unwired: 4 in]
                  }
                }
                n13 = call <vilib>:"Add State(s) to Queue__jki_lib_state_machine.vi"("State(s) in Front (\"\")"=w43, "State(s) in (\"\")"=w47) -> ("States Out"=w46:string)  [unwired: 13 in]
              }
              event #1 (no event record) {
                # "command you want to send to\nthe instrument process"
                n14 = event-data() -> ("OldVal"=w55)  [unwired: 1 in, 5 out]
                n15 = local write item#-1(w55) -> ()
                n16 = call <vilib>:"Build State String with Arguments__JKI_lib_State_Machine.vi"("Arguments (\"\")"="Command" ("State(s) in Front (\"\")"), "State"="Action: Command" ("State(s) in Front (\"\")")) -> ("State with Arguments"=w52:string)  [unwired: 4 in]
                n17 = call <vilib>:"Add State(s) to Queue__jki_lib_state_machine.vi"("State(s) in Front (\"\")"=w52, "State(s) in (\"\")"=w59) -> ("States Out"=w58:string)  [unwired: 13 in]
              }
              event #2 (no event record) {
                n18 = event-data() -> ("NewVal"=w62)  [unwired: 1 in, 5 out]
                n19 = Bundle By Name(cluster=w61, "Parameter"=w62) -> (w60:cluster{})
                n20 = call <vilib>:"Add State(s) to Queue__jki_lib_state_machine.vi"("State(s) in (\"\")"=w65) -> ("States Out"=w64:string)  [unwired: 14 in]
              }
              event Panel Close? {
                # "Discard the event because we'll close the front panel ourselves in Macro: Exit"
                # "Close Panel button (pressed) Event\n(this executes Macro: Exit to terminate the VI)"
                n21 = event-data() -> ()  [unwired: 1 in, 1 out]
                n22 = event-data("Discard?"=FALSE) -> ()  [unwired: 1 in, 1 out]
                n23 = call <vilib>:"Add State(s) to Queue__jki_lib_state_machine.vi"("State(s) in Front (\"\")"="Action: Notify UI Closed\nMacro: Exit", "State(s) in (\"\")"=w71) -> ("States Out"=w70:string)  [unwired: 13 in]
              }
              event User Event {
                n24 = event-data() -> ()  [unwired: 1 in, 5 out]
                n25 = call <vilib>:"Add State(s) to Queue__jki_lib_state_machine.vi"("State(s) in Front (\"\")"="Macro: Exit", "State(s) in (\"\")"=w76) -> ("States Out"=w75:string)  [unwired: 13 in]
              }
              event User Event {
                # "On Abort, no nice macro exit, but exit right away"
                n26 = event-data() -> ()  [unwired: 1 in, 5 out]
                n27 = call <vilib>:"Add State(s) to Queue__jki_lib_state_machine.vi"("State(s) in Front (\"\")"="Exit", "State(s) in (\"\")"=w81) -> ("States Out"=w80:string)  [unwired: 13 in]
              }
              event "STOP": Value Change {
                # "On Abort, no nice macro exit, but exit right away"
                n28 = event-data() -> ()  [unwired: 1 in, 6 out]
                n29 = Two Button Dialog(message="Are you sure you want to stop this program?") -> (T button?=w86:bool)  [unwired: 2 in]
                n30 = Select(t="Macro: Exit", s=w86, f="") -> (s? t:f=w82:string)
                n31 = call <vilib>:"Add State(s) to Queue__jki_lib_state_machine.vi"("State(s) in Front (\"\")"=w82, "State(s) in (\"\")"=w90) -> ("States Out"=w89:string)  [unwired: 13 in]
              }
            }
          }
          frame "---------- Core ----------" {
            # "Do not put any code in this frame.\n(it is a separator no-op)"
            n32 = call <vilib>:"Add State(s) to Queue__jki_lib_state_machine.vi"("State(s) in (\"\")"=w95) -> ("States Out"=w94:string)  [unwired: 14 in]
          }
          frame Default {
            w106 = 42 items=["No error", "Argument error", "Memory is full", "Out of zone", "End of file", "File already open", "Generic file I/O error", "File not found", "File permission error", "Disk is full", "Duplicate path", "Too many files open", "System feature not enabled", "Resource file not found", "Cannot add resource", "Resource not found", "Image not found", "Image memory error", "Pen does not exist", "Config type invalid", "Config token not found", "Config parse error", "Config memory error", "Bad external code format", "Bad external code offset", "External code not present", "Null window", "Destroy window error", "Null menu", "Print aborted", "Bad print record", "Print driver error", "Windows error during printing", "Memory error during printing", "Print dialog error", "Generic print error", "Invalid device refnum", "Device not found", "Device parameter error", "Device unit error", "Cannot open device", "Device call aborted", "Generic error", "Cancelled by user", "Object ID too low", "Object ID too high", "Object not in heap", "Unknown heap", "Unknown object (invalid DefProc)", "Unknown object (DefProc not in table)", "Message out of range", "Invalid (null) method", "Unknown message", "Manager call not supported", "Bad address", "Network operation in progress", "Network operation timed out", "Connection is busy", "Network attribute not supported", "Network error", "Address in use", "System out of memory", "Connection aborted", "Connection refused", "Not connected", "Already connected", "Connection closed", "Initialization error (interapplication manager)", "Bad occurrence", "Wait on unbound occurrence handler", "Occurrence queue overflow", "Datalog type conflict", "Unused", "Unrecognized type (interapplication manager)", "Memory corrupt", "Failed to make temporary DLL", "Old CIN version", "Drag socket not found", "Failed to load drop-object", "Failed to register OLE object", "Failed to release OLE object", "Format specifier type mismatch", "Unknown format specifier", "Too few format specifiers", "Too many format specifiers", "Scan failed", "Newer CIN version", "Error converting to variant", "Runtime menu error", "Password tampered", "Variant attribute not found", "Incompatible variant data type", "Event data is not available", "Event Store is not present", "Occurrence is not found", "Event Queue is not created", "Event info is not available", "Refnum passed is NULL", "Error retrieving Class GUID", "Error retrieving CoClass GUID", "Error retrieving TypeLib GUID.", "Bad built application magic bytes.", "Specific driver is different from the specific driver associated with the Logical Name.", "There is no session opened to the class driver.", "Max Error", "MAX - Error with config objects", "MAX - Error loading configuration", "MAX - Group not supported"]
            # "Current State"
            # "Do not delete, rename, or modify this frame.\n(this is used to capture unhandled states and typos)"
            # "Handle mistyped state name (developer tool)"
            n33 = Format Into String(format string="Software Exception: Unhandled State \"%s\"." ("message"), error in=w102, w97) -> (resulting string=w105:string, error out=w104:errorcluster)  [unwired: 1 in]
            n34 = call <vilib>:"Error Cluster From Error Code.vi"("show call chain? (False)"=TRUE, "error in (no error)"=w104, "error message (\"\")"=w105, "error code (0)"=w106) -> ("error out"=w103:errorcluster)  [unwired: 5 in]
            n35 = call <vilib>:"Add State(s) to Queue__jki_lib_state_machine.vi"("State(s) in (\"\")"=w101) -> ("States Out"=w100:string)  [unwired: 14 in]
          }
          frame "Initialize Core Data" {
            # "Do not delete, rename, or modify this frame.\n(this is used to determine panel behavior on exit)"
            # "originally closed?"
            # "exe?"
            # "If panel starts closed or is an EXE, then close it when we exit"
            n36 = property class="VI"() -> ("Front Panel.Open"=w116:bool)  [unwired: 2 in, 2 out]
            n37 = property class="App"() -> ("App.Kind"=w115:T23)  [unwired: 2 in, 2 out]
            n38 = control-ref of="Current VI Reference"() -> (w109:refnum<vi>)
            n39 = Not(x=w116) -> (.not. x?=w113:bool)
            n40 = Equal?(x=w115, y=T23."Run Time System" ("Application:Kind")) -> (x = y?=w112:bool)
            n41 = Or(x=w113, y=w112) -> (x .or. y?=w110:bool)
            n42 = Bundle By Name(cluster=w111, "Current VI Reference"=w109, "Close Panel on Exit?"=w110) -> (w118:cluster{})
            n43 = call <vilib>:"Add State(s) to Queue__jki_lib_state_machine.vi"("State(s) in (\"\")"=w120) -> ("States Out"=w119:string)  [unwired: 14 in]
          }
          frame "Error Handler" {
            w125 = errorcluster {"status"=FALSE, "code"=0, "source"=""}  # No error
            # "Overwrite this method to handle errors and pass to parent if not handled. Parent will fire a public event if the error is not handled up the chain of classes."
            # "Handle any errors here.\nYou can also output any states to clean-up after errors occur"
            n44 = Unbundle By Name(w123) -> ("Self Reference"=w131)
            n45 = call-dynamic "Handle Error.vi"("Stop on Unhandled Error (T)"=TRUE, "error in"=w130, "Instrument UI"=w131) -> ("handling error"=w126:errorcluster, "Unhandled error"=w124:errorcluster)  [unwired: 6 in, 1 out]
            n46 = Bundle By Name(cluster=w123, "error"=w124) -> (w122:cluster{})
            n47 = Select(t="Exit", s=w126, f="") -> (s? t:f=w127:string)
            n48 = call <vilib>:"Add State(s) to Queue__jki_lib_state_machine.vi"("State(s) in Front (\"\")"=w127, "State(s) in (\"\")"=w134) -> ("States Out"=w133:string)  [unwired: 13 in]
          }
          frame "Exit" {
            # "Do not put any code in this frame.\n(No errors that occur here will be handled.)"
            n49 = Unbundle By Name(w136) -> ("error"=w135)
            n50 = call <vilib>:"Add State(s) to Queue__jki_lib_state_machine.vi"("State(s) in (\"\")"=w140) -> ("States Out"=w139:string)  [unwired: 14 in]
          }
          frame "---------- Data ----------" {
            # "Do not put any code in this frame.\n(It is a separator no-op. You can make a copy of this frame to create a new Data frame)"
            n51 = call <vilib>:"Add State(s) to Queue__jki_lib_state_machine.vi"("State(s) in (\"\")"=w145) -> ("States Out"=w144:string)  [unwired: 14 in]
          }
          frame "Data: Initialize" {
            w147 = variant  # getAll
            w150 = T26 {"Current VI Reference"=refnum, "Close Panel on Exit?"=FALSE, "error"={"status"=FALSE, "code"=0, "source"=""}}  # Core
            w153 = refnum<class "Instrument.Lockin.UI.lvclass"> refnum  # Self Reference
            # "do not delete - used by framework"
            # "Data names and types of shift register data are defined by this bundle."
            # "Initialize the shift-register data, here.\n(data names are defined by what you wire into the bundle function)"
            n52 = Variant To Data(error in=w155, type=w153, Variant=w152) -> (data=w149:refnum<class "Instrument.Lockin.UI.lvclass">, error out=w154:errorcluster)
            n53 = Unbundle By Name(w149) -> ("Instrument"=w148:refnum<class "Instrument.lvclass">)
            n54 = Bundle("Core"=w150, "Self Reference"=w149, "Instrument"=w148, "getAll"=w147) -> (w156:T27, w146)  [unwired: 1 in]
            n55 = call <vilib>:"Add State(s) to Queue__jki_lib_state_machine.vi"("State(s) in (\"\")"=w158) -> ("States Out"=w157:string)  [unwired: 14 in]
          }
          frame "Data: Cleanup" {
            # "Cleanup any data and references, here.\n(this is called automatically, by the Macro: Exit)"
            n56 = Unbundle By Name(w160) -> ("Current VI Reference"=w163)
            n57 = Close Reference(reference=w163, error in (no error)=w162) -> (error out=w161:errorcluster)
            n58 = call <vilib>:"Add State(s) to Queue__jki_lib_state_machine.vi"("State(s) in (\"\")"=w165) -> ("States Out"=w164:string)  [unwired: 14 in]
          }
          frame "---------- UI ----------" {
            # "Do not put any code in this frame.\n(It is a separator no-op. You can make a copy of this frame to create a new UI frame)"
            n59 = call <vilib>:"Add State(s) to Queue__jki_lib_state_machine.vi"("State(s) in (\"\")"=w170) -> ("States Out"=w169:string)  [unwired: 14 in]
          }
          frame "UI: Initialize" {
            # "size window to decoration box on front panel"
            # "Initialize the User Interface, here.\n(this is called automatically, by the Macro: Init)"
            n60 = invoke on="STOP" class="Bool (strict)" method="Reinit To Default"() -> ()  [unwired: 3 in, 3 out]
            n61 = call <userlib>:"Fit VI window to Largest Dec__ogtk.vi"("error in (no error)"=w173, "border spacing (2 px)"=0) -> ("error out"=w172:errorcluster)  [unwired: 4 in, 1 out]
            n62 = call <vilib>:"Add State(s) to Queue__jki_lib_state_machine.vi"("State(s) in (\"\")"=w177) -> ("States Out"=w176:string)  [unwired: 14 in]
          }
          frame "UI: Cursor Set" {
            # "Argument"
            # "Initialize the User Interface, here.\n(this is called automatically, by the Macro: Init)"
            n63 = disable-structure shown="Default" {
              disable-tunnel: w180 -> [w185 w188]
              disable-tunnel: [w185 w187] -> w179
              disable-tunnel: w178 -> [_ w186]
              frame condition #0 {
              }
              frame condition #1 (active) {
                n64 = case shown="\"Busy\"" w186 {
                  tunnel: w188 -> [w190 w192]
                  tunnel: [w189 w191] -> w187
                  frame "Idle", Default {
                    n65 = call <vilib>:"Unset Busy.vi"("error in (no error)"=w190) -> ("error out"=w189:errorcluster)  [unwired: 10 in]
                  }
                  frame "Busy" {
                    n66 = call <vilib>:"Set Busy.vi"("error in (no error)"=w192) -> ("error out"=w191:errorcluster)  [unwired: 9 in, 1 out]
                  }
                }
              }
            }
            n67 = call <vilib>:"Add State(s) to Queue__jki_lib_state_machine.vi"("State(s) in (\"\")"=w184) -> ("States Out"=w183:string)  [unwired: 14 in]
          }
          frame "UI: Front Panel State" {
            # "Argument"
            # "Set Front Panel Open or Closed\n(Usage: \"UI: Front Panel State >> Open|Close\")"
            n68 = Unbundle By Name(w196) -> ("Current VI Reference"=w195)
            n69 = disable-structure shown="Default" {
              disable-tunnel: w198 -> [w204 w227]
              disable-tunnel: [w203 w227] -> w197
              disable-tunnel: w195 -> [w202 _]
              disable-tunnel: w194 -> [w201 _]
              frame condition #0 (active) {
                n70 = case shown="\"Close\"" w201 {
                  tunnel: w204 -> [w208 w221]
                  tunnel: [w210 w222] -> w203
                  tunnel: w202 -> [w209 w219]
                  frame "Open", Default {
                    n71 = property class="VI"(reference=w209, error in=w208) -> (reference out=w206:refnum<vi>, error out=w207:errorcluster, "FP.State"=w205:T24)
                    n72 = case shown="\"Closed\"" w205 {
                      tunnel: [w213 w216] -> w210
                      tunnel: w207 -> [w212 w216]
                      tunnel: w206 -> [w211 _]
                      frame "Closed" {
                        n73 = invoke class="VI" method="FP.Open"(reference=w211, error in=w212, "Activate"=TRUE, "State"=T24."Standard") -> (error out=w213:errorcluster)  [unwired: 1 in, 4 out]
                      }
                      frame Default {
                      }
                    }
                  }
                  frame "Close" {
                    n74 = property class="VI"(reference=w219, error in=w221) -> (reference out=w218:refnum<vi>, error out=w220:errorcluster, "FP.State"=w217:T24)
                    n75 = case shown="Default" w217 {
                      tunnel: [w223 w226] -> w222
                      tunnel: w220 -> [w223 w225]
                      tunnel: w218 -> [_ w224]
                      frame "Invalid", "Closed" {
                      }
                      frame Default {
                        n76 = invoke class="VI" method="FP.Close"(reference=w224, error in=w225) -> (error out=w226:errorcluster)  [unwired: 1 in, 2 out]
                      }
                    }
                  }
                }
              }
              frame condition #1 {
              }
            }
            n77 = call <vilib>:"Add State(s) to Queue__jki_lib_state_machine.vi"("State(s) in (\"\")"=w200) -> ("States Out"=w199:string)  [unwired: 14 in]
          }
          frame "---------- Macro ----------" {
            # "Do not put any code in this frame.\n(It is a separator no-op. You can make a copy of this frame to create a new Macro frame)"
            n78 = call <vilib>:"Add State(s) to Queue__jki_lib_state_machine.vi"("State(s) in (\"\")"=w232) -> ("States Out"=w231:string)  [unwired: 14 in]
          }
          frame "Macro: Initialize" {
            w235 = "UI: Initialize\n//UI: Front Panel State >> Open"  # UI: Initialize //UI: Front Panel State >> Open
            # "Initialization Macro\n(This is called once, when the VI starts)"
            n79 = call <vilib>:"Add State(s) to Queue__jki_lib_state_machine.vi"("State(s) in Front (\"\")"="Data: Initialize\nInitialize Core Data\nEvents: Register", "State(s) in (\"\")"="Process: Sync", "State(s) at Back (\"\")"=w235) -> ("States Out"=w234:string)  [unwired: 12 in]
            n80 = call <vilib>:"Add State(s) to Queue__jki_lib_state_machine.vi"("State(s) in Front (\"\")"=w234, "State(s) in (\"\")"=w241) -> ("States Out"=w240:string)  [unwired: 13 in]
          }
          frame "Macro: Exit" {
            # "Exit Macro\n(This is called once, when the VI exits)"
            n81 = Unbundle By Name(w246) -> ("Close Panel on Exit?"=w252)
            n82 = Select(t="//UI: Front Panel State >> Close", s=w252, f="") -> (s? t:f=w249:string)
            n83 = call <vilib>:"Add State(s) to Queue__jki_lib_state_machine.vi"("State(s) in Front (\"\")"="Data: Cleanup\nEvents: Unregister\nProcess: Self Terminate", "State(s) in (\"\")"="Process: Sync", "State(s) at Back (\"\")"="Exit") -> ("States Out"=w243:string)  [unwired: 12 in]
            n84 = call <vilib>:"Add State(s) to Queue__jki_lib_state_machine.vi"("State(s) in (\"\")"=w249, "State(s) at Back (\"\")"=w243) -> ("States Out"=w248:string)  [unwired: 13 in]
            n85 = call <vilib>:"Add State(s) to Queue__jki_lib_state_machine.vi"("State(s) in Front (\"\")"=w248, "State(s) in (\"\")"=w255) -> ("States Out"=w254:string)  [unwired: 13 in]
          }
          frame "---------- Process ----------" {
            # "Template Separator\n(You can make a copy of, or modify, this frame)"
            n86 = call <vilib>:"Add State(s) to Queue__jki_lib_state_machine.vi"("State(s) in (\"\")"=w260) -> ("States Out"=w259:string)  [unwired: 14 in]
          }
          frame "Process: Sync" {
            n87 = Unbundle By Name(w268) -> ("Self Reference"=w264)
            n88 = call <vilib>:"WaitOnProcessSync.vi"("error in (no error)"=w263, "SMO"=w264) -> ("error out"=w262:errorcluster, "Don't run?"=w267:bool)  [unwired: 7 in, 1 out]
            n89 = Select(t="Data: Cleanup\nEvents: Unregister\nExit", s=w267, f="") -> (s? t:f=w261:string)
            n90 = call <vilib>:"Add State(s) to Queue__jki_lib_state_machine.vi"("State(s) in Front (\"\")"=w261, "State(s) in (\"\")"=w271) -> ("States Out"=w270:string)  [unwired: 13 in]
          }
          frame "Process: Self Terminate" {
            n91 = Unbundle By Name(w273) -> ("Self Reference"=w272)
            n92 = call <vilib>:"SelfTerminate.vi"("error in (no error)"=w275, "SMO in"=w272) -> ("error out"=w274:errorcluster)  [unwired: 8 in, 1 out]
            n93 = call <vilib>:"Add State(s) to Queue__jki_lib_state_machine.vi"("State(s) in (\"\")"=w278) -> ("States Out"=w277:string)  [unwired: 14 in]
          }
          frame "---------- Events ----------" {
            # "Template Separator\n(You can make a copy of, or modify, this frame)"
            n94 = call <vilib>:"Add State(s) to Queue__jki_lib_state_machine.vi"("State(s) in (\"\")"=w283) -> ("States Out"=w282:string)  [unwired: 14 in]
          }
          frame "Events: Register" {
            # "Expand to add\nmore events"
            # "Base Class Protected Events"
            n95 = Unbundle By Name(w294) -> ("Self Reference"=w287, "Instrument"=w286)
            n96 = call <vilib>:"GetProtectedEvents.vi"("SMO"=w287) -> ("error out"=w288:errorcluster, "SMO Protected Events"=w292:T28)  [unwired: 8 in, 1 out]
            n97 = call <userlib>:"Instrument.GetPublicEvents.vi"("Instrument"=w286) -> ("error out"=w284:errorcluster, "Instrument Public Events"=w285:T29)  [unwired: 8 in, 1 out]
            n98 = register-events(w292, w285) -> (reference out=w293:refnum<event-registration>, error out=w290:errorcluster)  [unwired: 2 in]
            n99 = Merge Errors(w284, w291, w290, w288) -> (w289:errorcluster)
            n100 = call <vilib>:"Add State(s) to Queue__jki_lib_state_machine.vi"("State(s) in (\"\")"=w296) -> ("States Out"=w295:string)  [unwired: 14 in]
          }
          frame "Events: Unregister" {
            n101 = Unregister For Events(event registration refnum=w299, error in=w298) -> (error out=w297:errorcluster)
            n102 = call <vilib>:"Add State(s) to Queue__jki_lib_state_machine.vi"("State(s) in (\"\")"=w302) -> ("States Out"=w301:string)  [unwired: 14 in]
          }
          frame "---------- Action ----------" {
            n103 = Unbundle By Name(w305) -> ("Self Reference"=w303)
            n104 = Bundle By Name(cluster=w305, "Self Reference"=w303) -> (w304:cluster{})
            n105 = call <vilib>:"Add State(s) to Queue__jki_lib_state_machine.vi"("State(s) in (\"\")"=w309) -> ("States Out"=w308:string)  [unwired: 14 in]
          }
          frame "Action: Notify UI Closed" {
            # "Notify that the UI has been closed"
            n106 = Unbundle By Name(w312) -> ("Self Reference"=w313)
            n107 = call <vilib>:"Hide.vi"("error in (no error)"=w311, "SMO.UI"=w313) -> ("error out"=w310:errorcluster)  [unwired: 8 in, 1 out]
            n108 = call <vilib>:"Add State(s) to Queue__jki_lib_state_machine.vi"("State(s) in (\"\")"=w316) -> ("States Out"=w315:string)  [unwired: 14 in]
          }
          frame "Action: Update Front Panel" {
            # "do this way to have nicer UI or only display what you want"
            # "typedef from Child Instrument"
            n109 = Unbundle By Name(w323) -> ("getAll"=w322)
            n110 = Variant To Data(error in=w320, type=T25 {"Not Supported"=""} ("getAll"), Variant=w322) -> (data=w318:T25, error out=w319:errorcluster)
            n111 = Unbundle By Name(w318) -> ("Not Supported"=w317:string)
            n112 = call <vilib>:"Add State(s) to Queue__jki_lib_state_machine.vi"("State(s) in (\"\")"=w326) -> ("States Out"=w325:string)  [unwired: 14 in]
          }
          frame "Action: Command" {
            # "#todo:\nconfigure here how to parse messages from Instrument"
            # "command"
            n113 = Unbundle By Name(w338) -> ("Self Reference"=w331, "Instrument"=w329, "Parameter"=w336)
            n114 = case shown="\"setMagnet\"" w333 {
              tunnel: w336 -> [_ w348 w360]
              tunnel: w335 -> [w346 w351 w358]
              tunnel: [w346 w351 w356] -> w334
              tunnel: [w344 w350 w355] -> w332
              tunnel: w331 -> [w344 w350 w355]
              tunnel: ["" ("State(s) in Front (\"\")") "Action: Update Front Panel" ("State(s) in Front (\"\")") "" ("State(s) in Front (\"\")")] -> w330
              tunnel: w329 -> [w345 w347 w353]
              tunnel: [w345 w347 w353] -> w328
              tunnel: [variant ("Data out") w348 variant ("Data out")] -> w327
              frame Default {
              }
              frame "getAll" {
              }
              frame "setMagnet" {
                n115 = Variant To Data(error in=w358, type=0.0 ("Magnet Return"), Variant=w360) -> (data=w357:dbl, error out=w356:errorcluster)
              }
            }
            n116 = Bundle By Name(cluster=w338, "Self Reference"=w332, "Instrument"=w328, "getAll"=w327) -> (w337:cluster{})
            n117 = call <vilib>:"Add State(s) to Queue__jki_lib_state_machine.vi"("State(s) in Front (\"\")"=w330, "State(s) in (\"\")"=w341) -> ("States Out"=w340:string)  [unwired: 13 in]
          }
        }
      }
    }
    frame Error {
    }
  }
  n118 = call-parent "Process.vi"("error in"=w8, "Instrument UI in"=w7) -> ("error out"=w5:errorcluster, "Instrument UI out"=→"Lockin.UI out":refnum<class "Instrument.Lockin.UI.lvclass">)  [unwired: 8 in]
  n119 = Merge Errors(w5, w4) -> (→"error out":errorcluster)
